vi "HIOKI PW3390 Motor 0Adjust.vi"(0 "VISA Resource":refnum<visa-resource-name>, 11 "error in (no error)":errorcluster, 13 "Error Out (F: Off)":bool) -> (4 "VISA Resource out":refnum<visa-resource-name>, 15 "error out":errorcluster)   [LabVIEW 2009]
doc: "Executes zero adjust of Motor Analysis Option."
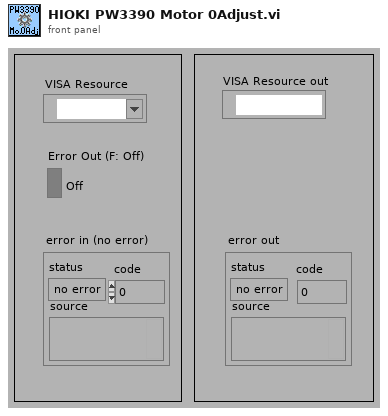
[diagram p1: front panel]
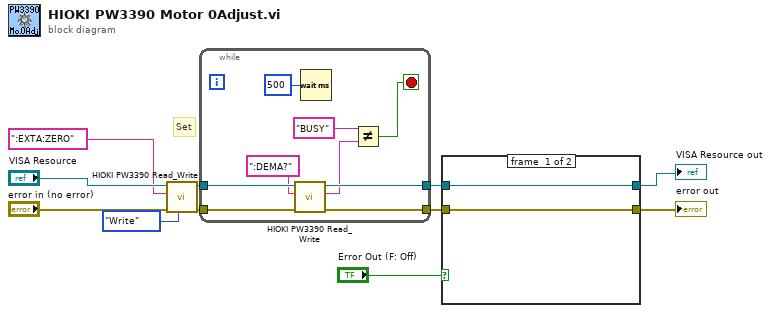
[diagram p0: block diagram]
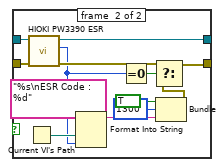
[diagram p2: hidden frame]
diagram:
  # "Set"
  n1 = call <instrlib>:"HIOKI PW3390 Read_Write.vi"("Read/Write"=enum16{"Read", "Write"}."Write", "error in (no error)"="error in (no error)", "data in"=":EXTA:ZERO", "VISA Resource"="VISA Resource") -> ("error out"=w1:errorcluster, "VISA Resource out"=w2:refnum<visa-resource-name>)  [unwired: 5 in, 1 out]
  n2 = while {
    tunnel: w2 -> [w19]
    tunnel: [w16] -> w4
    tunnel: w1 -> [w18]
    tunnel: [w15] -> w3
    stop <- w14 stop-if-true
    n3 = call <instrlib>:"HIOKI PW3390 Read_Write.vi"("error in (no error)"=w18, "data in"=":DEMA?", "VISA Resource"=w19) -> ("error out"=w15:errorcluster, "data out"=w13:string, "VISA Resource out"=w16:refnum<visa-resource-name>)  [unwired: 6 in]
    n4 = Wait (ms)(milliseconds to wait=u32 500) -> ()  [unwired: 1 out]
    n5 = Not Equal?(x="BUSY", y=w13) -> (x != y?=w14:bool)
  }
  n6 = case shown="TRUE" "Error Out (F: Off)" {
    tunnel: w4 -> [w22 w35]
    tunnel: w3 -> [w21 w34]
    tunnel: [w21 w24] -> w8
    tunnel: [w22 w33] -> w5
    frame #0 {
    }
    frame #1 {
      n7 = Current VI's Path() -> (path=w31:path)
      n8 = call <instrlib>:"HIOKI PW3390 ESR.vi"("error in (no error)"=w34, "VISA Resource"=w35) -> ("error out"=w25:errorcluster, "Output Value"=w23:u8, "VISA Resource out"=w33:refnum<visa-resource-name>)  [unwired: 6 in, 1 out]
      n9 = Format Into String(format string="%s\nESR Code : %d", w31, w23) -> (resulting string=w27:string)  [unwired: 2 in, 1 out]
      n10 = Equal To 0?(x=w23) -> (x = 0?=w32:bool)
      n11 = Bundle("status"=TRUE, "code"=1300, w27) -> (w26:cluster{"status":bool, "code":i32, string})  [unwired: 1 in]
      n12 = Select(t=w25, s=w32, f=w26) -> (s? t:f=w24:errorcluster)
    }
  }
  "error out" <- w8
  "VISA Resource out" <- w5
